vi "LVFunction_Imop_Check_ClosedLoopSecurity_HighLevel.vi"(5 "HasoSlopes in":refnum<class "HasoSlopes.lvclass">, 7 "CorrectionDataManager":refnum<class "CorrectionDataManager.lvclass">, 9 "CurrentPosition":T2, 11 "error IO":errorcluster, 13 "Fill Percent":sgl, 14 "DeltaPosition":T2) -> (6 "ClosedLoopSecurityActivationParams":T1, 15 "error IO out":errorcluster)   [LabVIEW 2020]
doc: "Compute slopes from modal coefficients that represent them in a given basis of\npolynomials provided by ComputePhaseSet.\n\n--------------------------------------------------------------------------------\n\nTypePhaseIn\n TypePhase Polynomial bases enumeration.\n\nTypePhaseOut\n TypePhase Polynomial bases enumeration.\n\nslopes\n cHasoSlopes object.\n\nComputePhaseSet\n cComputePhaseSet object.\n\ncoefs\n cModalCoef object.\n\nErrorIn\n Error\nErrorOut\n Error"
uses:
  CorrectionDataManager.lvclass
  Wavefront Corrector Position.ctl
  HasoSlopes.lvclass
  ClosedLoopSecurityActivationResults.ctl
  LVClass_HasoSlopes Read HasoSlopes _ property.vi
  LVClass_CorrectionDataManager Read CorrectionDataManager.vi
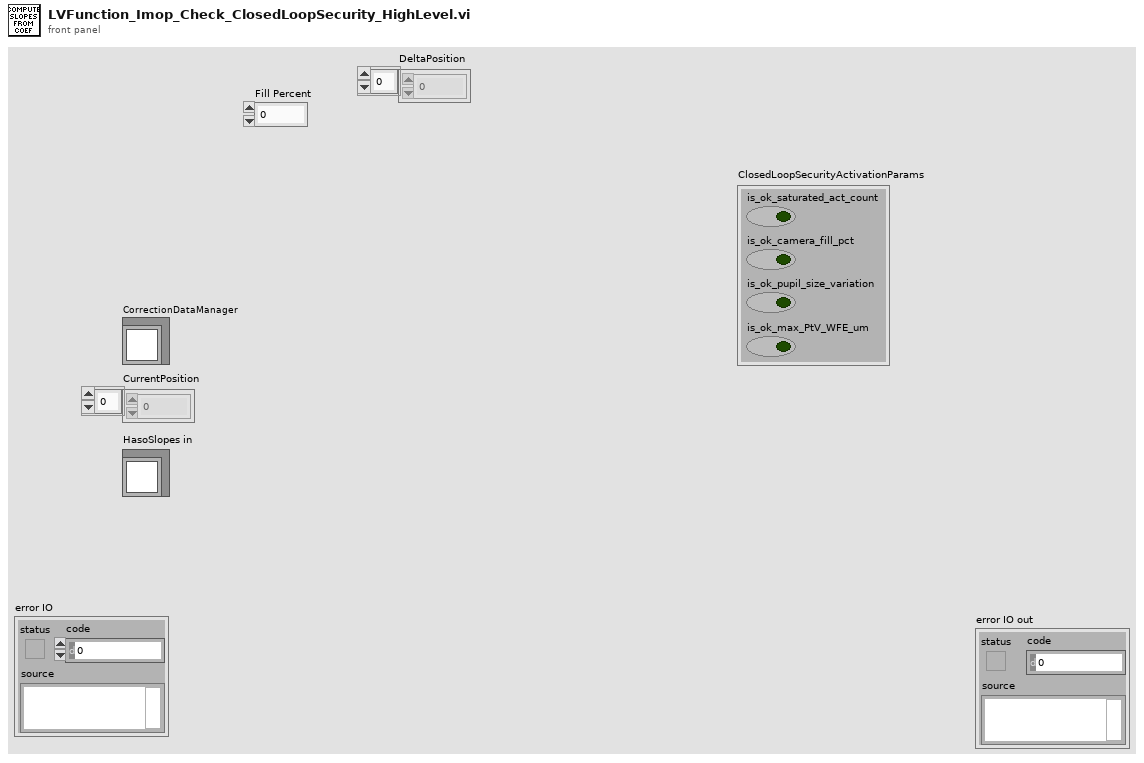
[diagram p1: front panel]
types:
  T1 = typedef "ClosedLoopSecurityActivationResults.ctl" = cluster{"is_ok_saturated_act_count":bool, "is_ok_camera_fill_pct":bool, "is_ok_pupil_size_variation":bool, "is_ok_max_PtV_WFE_um":bool}
  T2 = typedef "Wavefront Corrector Position.ctl" = sgl[]
  T3 = typedef "ClassID.ctl" = i64
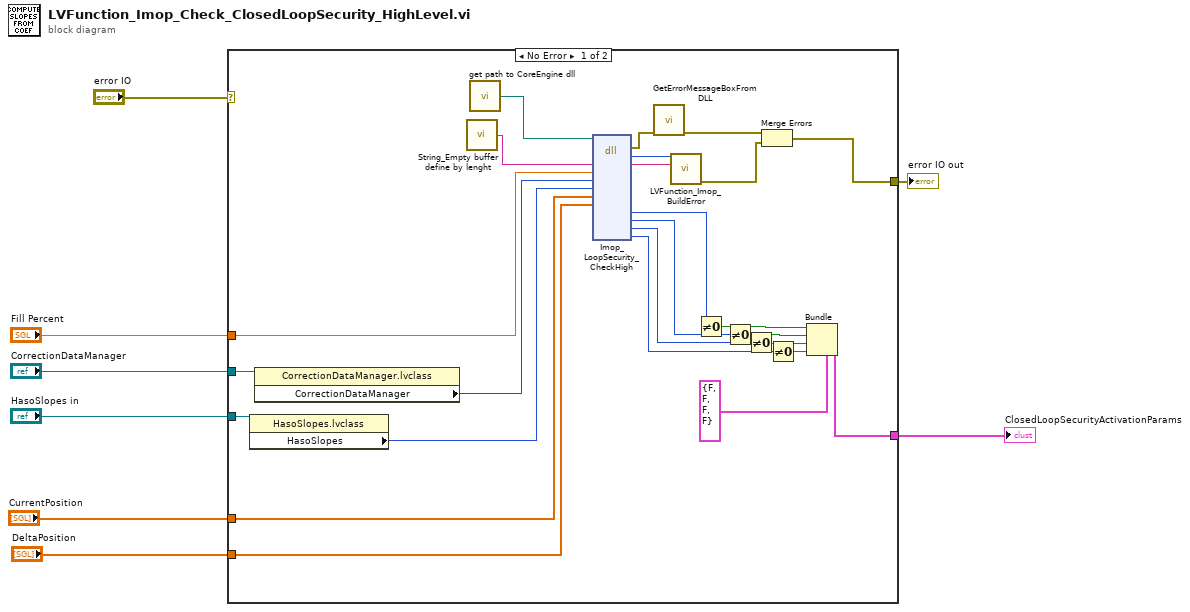
[diagram p0: block diagram]
diagram:
  n1 = case shown="No Error" "error IO" {
    selector: "error IO" -> [_ w34]
    tunnel: [w26 w34] -> w7
    tunnel: "CorrectionDataManager" -> [w25 _]
    tunnel: "Fill Percent" -> [w23 _]
    tunnel: "HasoSlopes in" -> [w24 _]
    tunnel: "CurrentPosition" -> [w9 _]
    tunnel: "DeltaPosition" -> [w20 _]
    tunnel: [w11 _] -> w1
    frame No Error {
      n2 = property class="HasoSlopes.lvclass"(reference=w24) -> ("HasoSlopes"=w21:T3)  [unwired: 1 in, 2 out]
      n3 = property class="CorrectionDataManager.lvclass"(reference=w25) -> ("CorrectionDataManager"=w22:T3)  [unwired: 1 in, 2 out]
      n4 = call "String_Empty buffer define by lenght.vi"() -> ("Empty buffer"=w31:string)  [unwired: 1 in]
      n5 = call "get path to CoreEngine dll.vi"() -> ("path to wavekit library"=w30:path)  [unwired: 14 in, 1 out]
      n6 = dll-call lib="D:/soft/HASO_v3/SVN_trunk/ImOpCoreEngine4_LV2011/DLLs/c_interface_vc100.dll" fn="Imop_LoopSecurity_CheckHigh"(path in=w30, "message"=w31, "camera_fill_percentage"=w23, "correction_data_manager"=w22, "delta_slopes_pupil"=w21, "Current_Commands"=w9, "delta_commands"=w20) -> (error out=w29:errorcluster, "return type"=w33:i32, "message"=w32:string, "is_ok_saturated_act_count"=w15:u8, "is_ok_camera_fill_pct"=w14:u8, "is_ok_pupil_size_variation"=w13:u8, "is_ok_loop_gain"=w12:u8)  [unwired: 11 in, 1 out]
      n7 = call "GetErrorMessageBoxFromDLL.vi"("error IN"=w29) -> ("error OUT"=w28:errorcluster)  [unwired: 10 in]
      n8 = call "LVFunction_Imop_BuildError.vi"("code"=w33, "String to Prepend to source (\"\")"=w32) -> ("error out"=w27:errorcluster)  [unwired: 13 in]
      n9 = Not Equal To 0?(x=w15) -> (x != 0?=w19:bool)
      n10 = Not Equal To 0?(x=w14) -> (x != 0?=w18:bool)
      n11 = Not Equal To 0?(x=w13) -> (x != 0?=w17:bool)
      n12 = Merge Errors(w28, w27) -> (w26:errorcluster)
      n13 = Not Equal To 0?(x=w12) -> (x != 0?=w16:bool)
      n14 = Bundle(cluster=T1 {"is_ok_saturated_act_count"=FALSE, "is_ok_camera_fill_pct"=FALSE, "is_ok_pupil_size_variation"=FALSE, "is_ok_max_PtV_WFE_um"=FALSE} ("ClosedLoopSecurityActivationParams"), "is_ok_saturated_act_count"=w19, "is_ok_camera_fill_pct"=w18, "is_ok_pupil_size_variation"=w17, "is_ok_max_PtV_WFE_um"=w16) -> (w11:T1)
    }
    frame Error {
    }
  }
  "error IO out" <- w7
  "ClosedLoopSecurityActivationParams" <- w1
